vi "Stop Motor.vi"(8 "error in (no error)":errorcluster, 11 "VacuumLine in":refnum<class "VacuumLine.lvclass">) -> (0 "error out":errorcluster, 3 "VacuumLine out":refnum<class "VacuumLine.lvclass">)   [LabVIEW 2016, in "Hardware.lvlib" / "VacuumLine.lvlib" / "VacuumLine.lvclass"]
uses:
  <userlib>/Common Components/Hardware/Abstract System/VacuumLine/VacuumLine/VacuumLine.lvclass
  <userlib>/Common Components/Hardware/Abstract System/VacuumLine/VacuumLine/VacuumLine.lvclass/VacuumLine.ctl
  <userlib>/Common Components/Hardware/Motor/Motor/Motor.lvclass
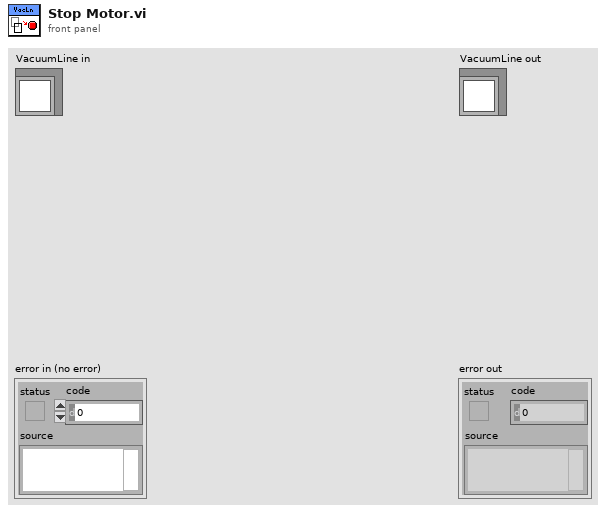
[diagram p1: front panel]
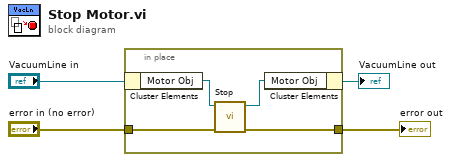
[diagram p0: block diagram]
diagram:
  n1 = in-place {
    in-place-border: "error in (no error)" -> [w8]
    in-place-border: [w7] -> w3
    n2 = in-place-cluster #1("VacuumLine in") -> ("Motor Obj"=w6:refnum<class "Motor.lvclass">)
    n3 = call-dynamic "Stop.vi"("error in (no error)"=w8, "Motor in"=w6) -> ("error out"=w7:errorcluster, "Motor out"=w5:refnum<class "Motor.lvclass">)  [unwired: 8 in]
    n4 = in-place-cluster #1("Motor Obj"=w5) -> (→"VacuumLine out":refnum<class "VacuumLine.lvclass">)
  }
  "error out" <- w3
